vi "PIDPressure2.vi"() -> ()   [LabVIEW 2015]
uses:
  <vilib>/DAQmx/write.llb/DAQmx Write (Digital 1D Bool NChan 1Samp 1Line).vi
  <vilib>/DAQmx/write.llb/DAQmx Write (Digital Bool 1Line 1Point).vi
  <vilib>/DAQmx/read.llb/DAQmx Read (Analog DBL 1Chan 1Samp).vi
  <vilib>/DAQmx/write.llb/DAQmx Write (Analog DBL 1Chan 1Samp).vi
  <vilib>/Analysis/baseanly.llb/Mean (DBL).vi
  <vilib>/DAQmx/read.llb/DAQmx Read (Analog 1D Wfm NChan NSamp).vi
  <vilib>/DAQmx/miscellaneous.llb/DAQmx Fill In Error Info.vi
  <vilib>/addons/control/pid/NI_PID_autopid.lvlib
  <vilib>/Analysis/NI_AALBase.lvlib
panel:
  in  "Manual Control 2":bool
  in  "Heater On/Off":bool
  out "Voltage Reading(Temp)":dbl format="%#_13g"
  out "Temperature (Celcius)":dbl format="%#.1g"
  out "Temp(C)":dbl(slide) scale=-10.0..100.0
  out "Temp Chart":dbl(graph)
  out "Temp Chart 2":dbl(graph)
  out "Temp":dbl
  in  "stop 2":bool
  in  "autotuning parameters 2":T1={"controller type"=1, "relay cycles"=3, "relay amplitude"=1.0, "control specification"=2, "PV noise level"=0.1} {"PV noise level" format="%.2f"; "control specification" items=["normal", "fast", "slow"]; "relay amplitude" format="%.2f"; "controller type" items=["PID", "PI", "P"]}
  in  "PID gains 2":T2={"proportional gain (Kc)"=1.0, "integral time (Ti, min)"=0.01, "derivative time (Td, min)"=0.0} {"derivative time (Td, min)" format="%.3f"; "integral time (Ti, min)" format="%.3f"; "proportional gain (Kc)" format="%.3f"}
  out "PID gains out 2":T2={"proportional gain (Kc)"=1.0, "integral time (Ti, min)"=0.01, "derivative time (Td, min)"=0.0} {"derivative time (Td, min)" format="%.3f"; "integral time (Ti, min)" format="%.3f"; "proportional gain (Kc)" format="%.3f"}
  in  "autotune? (F) 2":bool
  in  "reinitialize? (F) 2":bool
  in  "setpoint in C":dbl format="%.2f"
  out "Control Value Temp":dbl
  out "ms to wait":dbl
  out "Loop 1":i32
  out "Loop 2":i32
  in  "Voltage setting":dbl format="%#_13g"
  in  "Manual Control":bool
  out "Control Value":dbl
  in  "setpoint in Bar":dbl format="%#.5f"
  in  "reinitialize? (F)":bool
  in  "autotune? (F)":bool
  out "PID gains out":T2={"proportional gain (Kc)"=1.0, "integral time (Ti, min)"=0.01, "derivative time (Td, min)"=0.0} {"derivative time (Td, min)" format="%.3f"; "integral time (Ti, min)" format="%.3f"; "proportional gain (Kc)" format="%.3f"}
  in  "PID gains":T2={"proportional gain (Kc)"=1.0, "integral time (Ti, min)"=0.01, "derivative time (Td, min)"=0.0} {"derivative time (Td, min)" format="%.3f"; "integral time (Ti, min)" format="%.3f"; "proportional gain (Kc)" format="%.3f"}
  in  "autotuning parameters":T1={"controller type"=1, "relay cycles"=3, "relay amplitude"=1.0, "control specification"=2, "PV noise level"=0.1} {"PV noise level" format="%.2f"; "control specification" items=["normal", "fast", "slow"]; "relay amplitude" format="%.2f"; "controller type" items=["PID", "PI", "P"]}
  in  "stop":bool
  out "Pressure Chart 2":dbl(graph)
  out "Voltage":dbl(graph)
  out "Pressure":dbl format="%#.3g"
  out "Voltage Reading(pressure)":dbl format="%#_13g"
  # "Readings"
  # "Controls"
  # "PID Settings"
  # "51.12139\n\n0.044676"
  # "Readings"
  # "Controls"
  # "PID Settings"
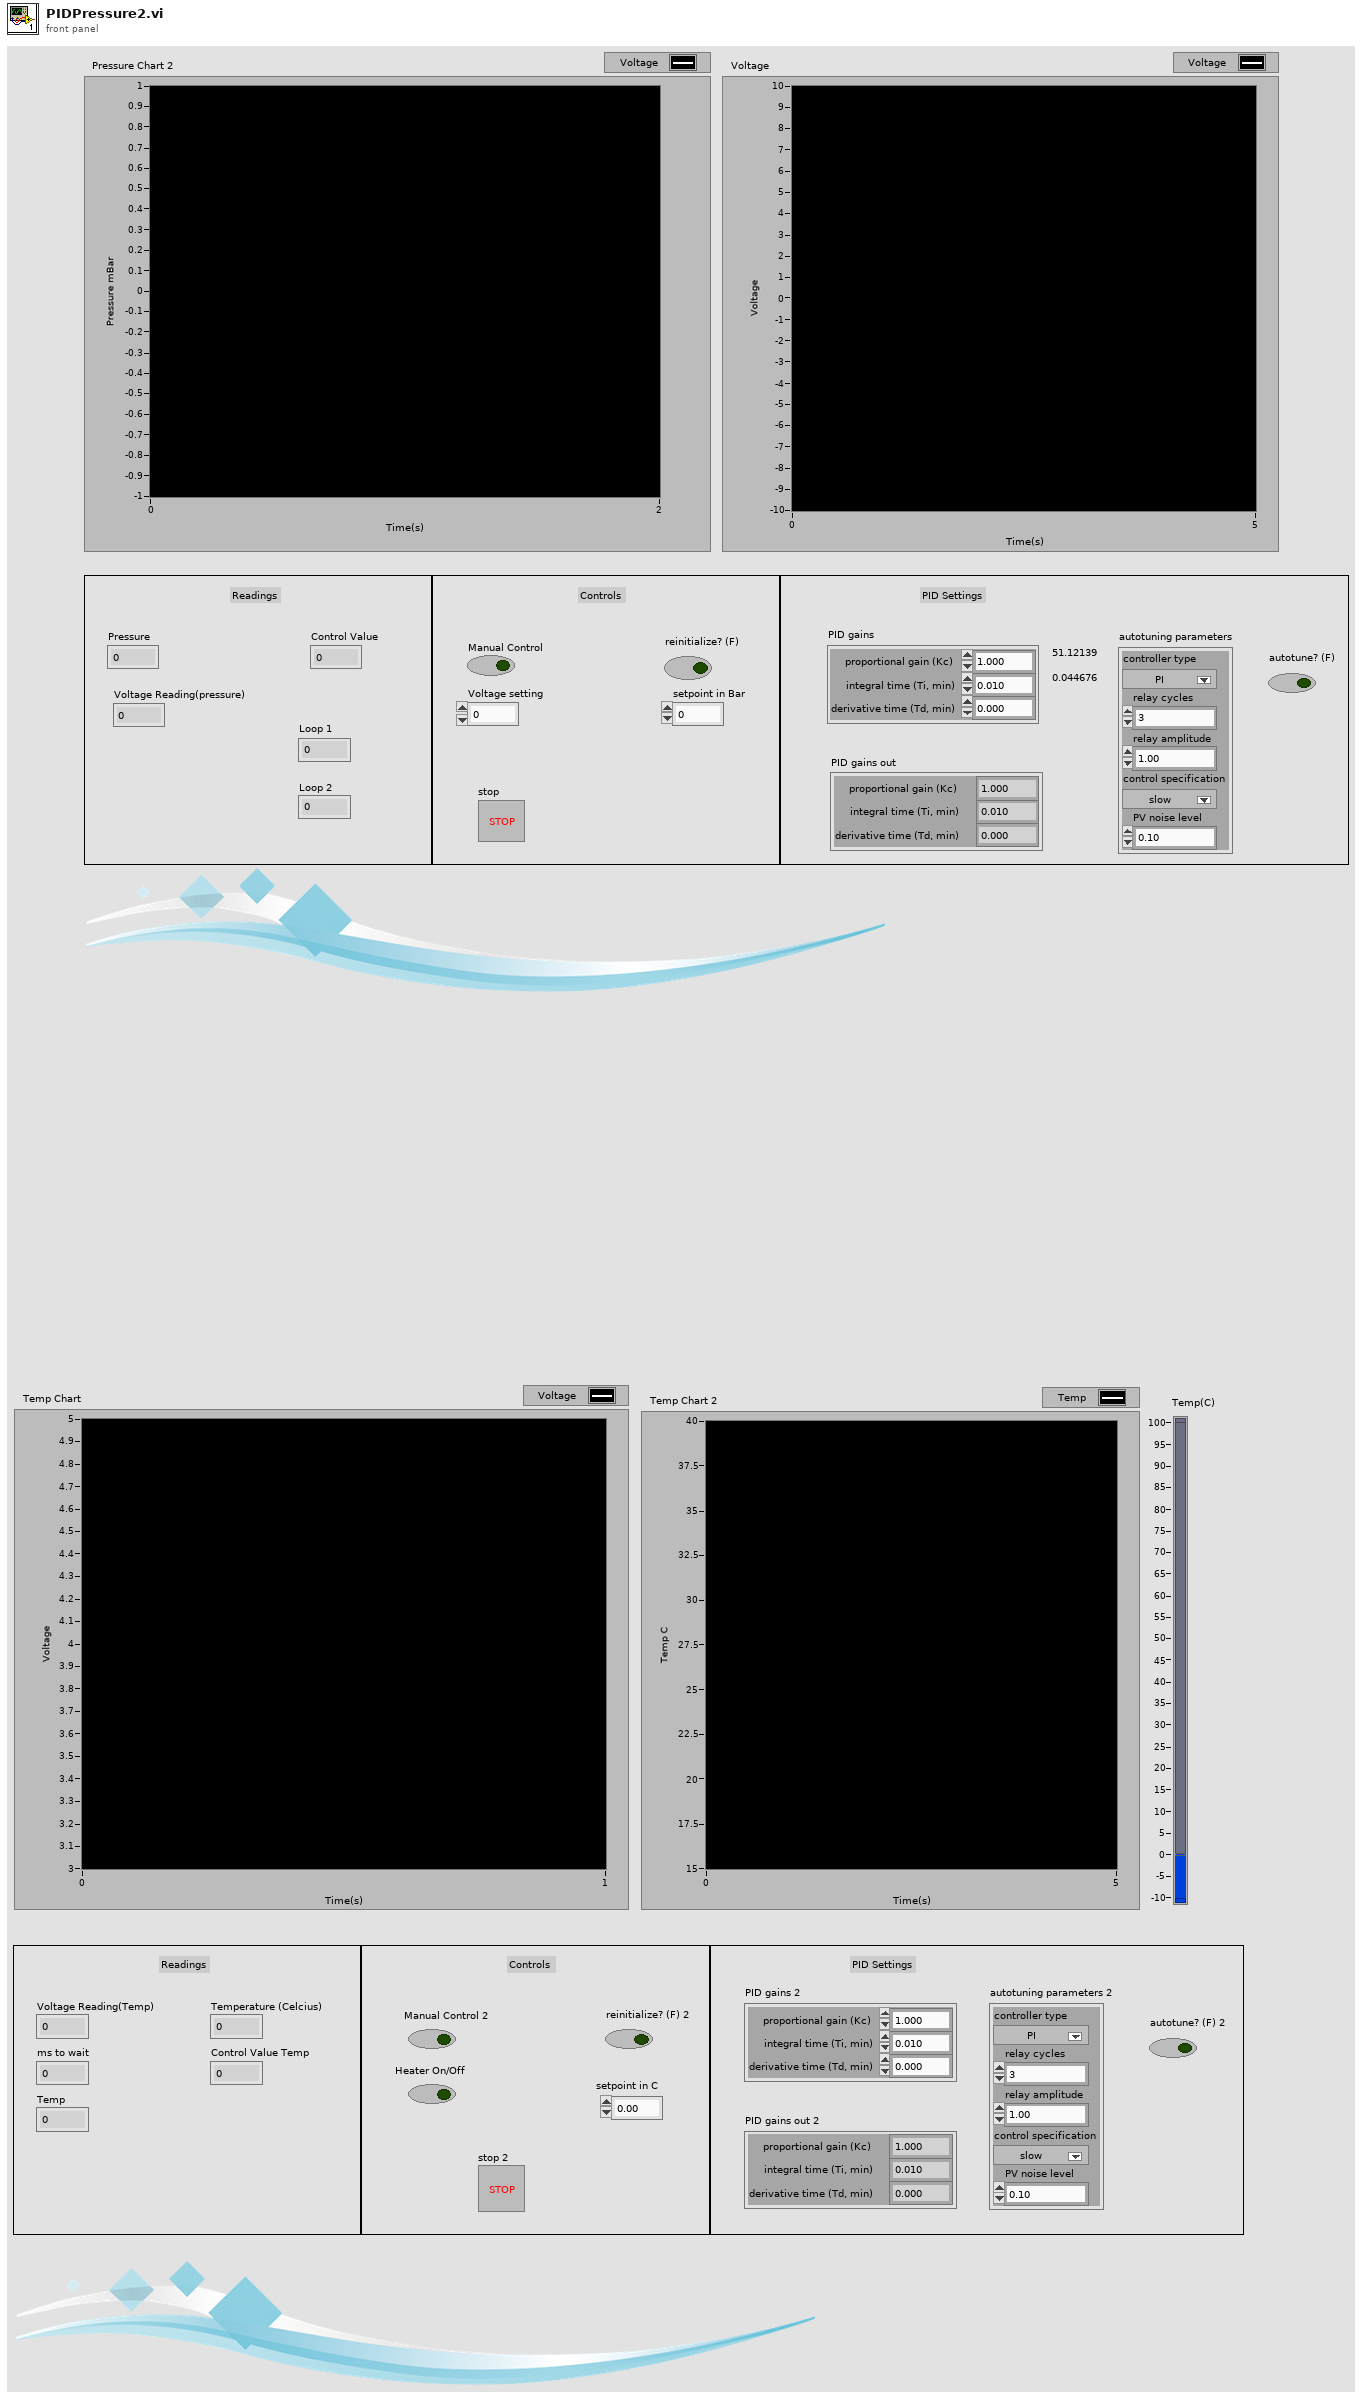
[diagram p1: front panel]
types:
  T1 = cluster{"controller type":u16, "relay cycles":i32, "relay amplitude":dbl, "control specification":u16, "PV noise level":dbl}
  T2 = cluster{"proportional gain (Kc)":dbl, "integral time (Ti, min)":dbl, "derivative time (Td, min)":dbl}
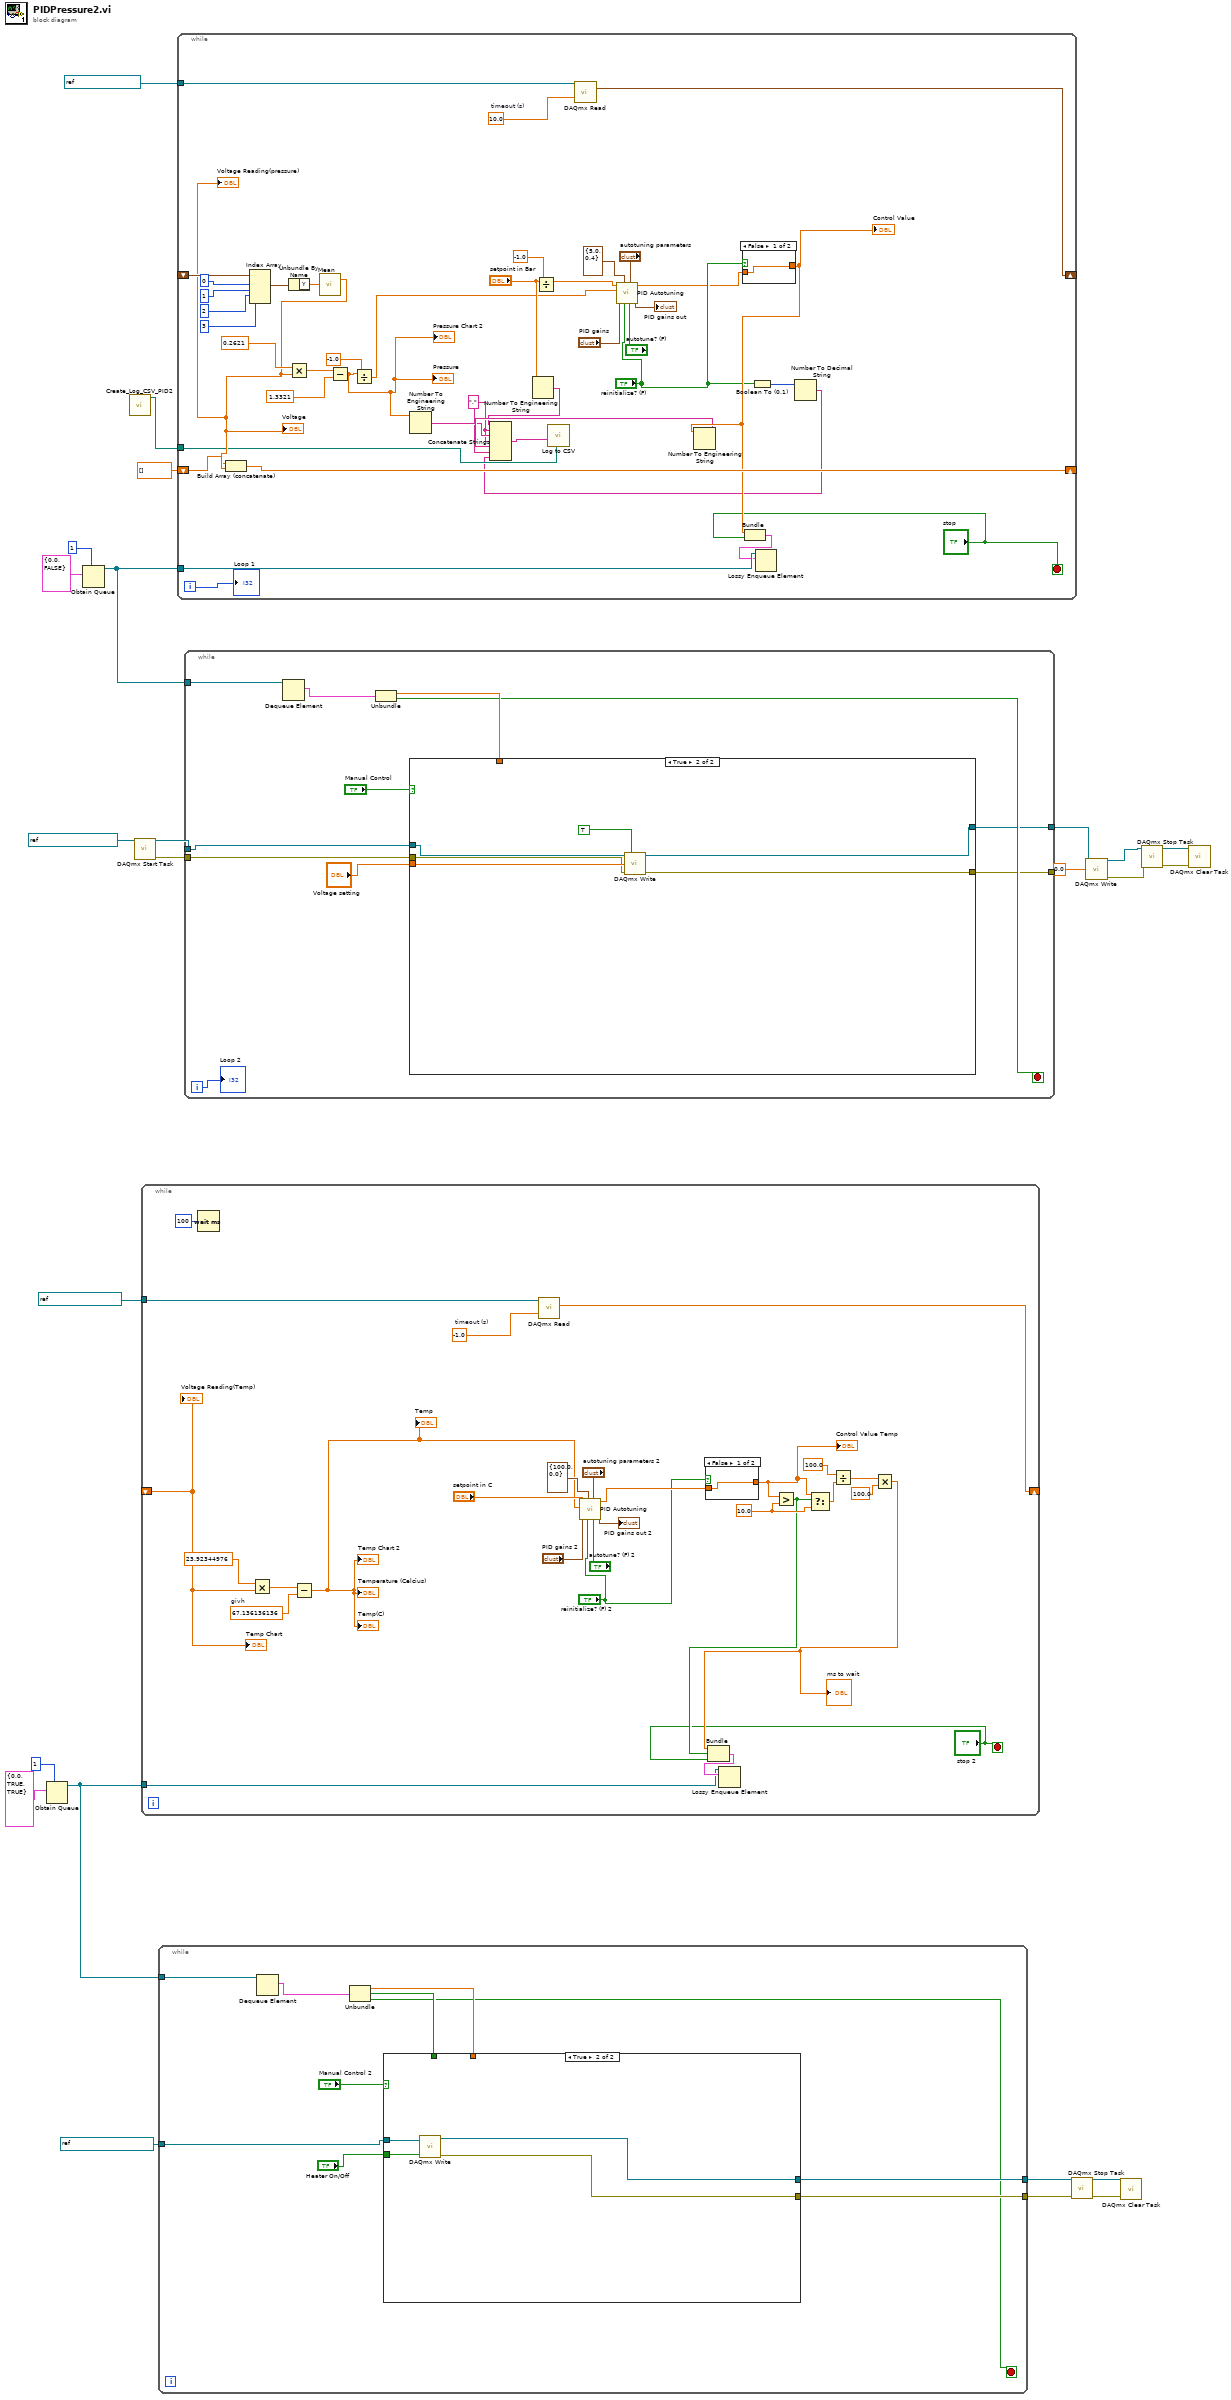
[diagram p0: block diagram]
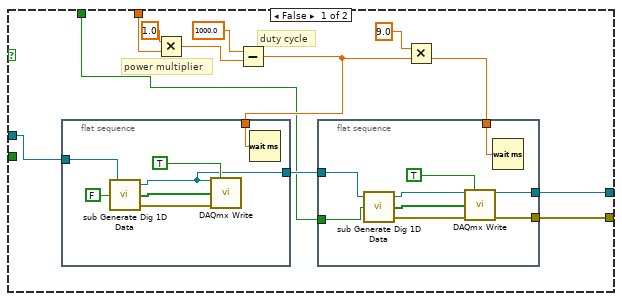
[diagram p2: hidden frame]
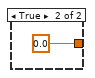
[diagram p3: hidden frame]
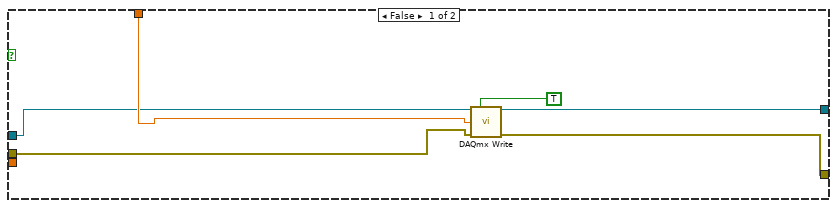
[diagram p4: hidden frame]
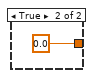
[diagram p5: hidden frame]
diagram:
  n1 = Obtain Queue(max queue size (-1, unlimited)=1, element data type=cluster{dbl, bool, bool} {0.0, TRUE, TRUE}) -> (queue out=w1:refnum<queue>)  [unwired: 3 in, 2 out]
  n2 = Obtain Queue(max queue size (-1, unlimited)=1, element data type=cluster{dbl, bool} {0.0, FALSE}) -> (queue out=w22:refnum<queue>)  [unwired: 3 in, 2 out]
  n3 = call "Create_Log_CSV_PID2.vi"() -> ("path"=w18:path)  [unwired: 11 in]
  n4 = call <vilib>:"DAQmx Start Task.vi"("task/channels in"=refnum<k21> "MyVoltageOutTask") -> ("task out"=w17:refnum<k21>, "error out"=w16:errorcluster)  [unwired: 13 in]
  n5 = while {
    tunnel: refnum<k21> "MyVoltageTask_0" -> [w48]
    shift-right: [w31] -> _
    shift-left: _ -> [w32]
    tunnel: w1 -> [w26]
    stop <- "stop 2" stop-if-true
    w34 = 10.0 ("f")
    w49 = 67.136136136  # givh
    w52 = -1.0  # timeout (s)
    n6 = Wait (ms)(milliseconds to wait=u32 100) -> ()  [unwired: 1 out]
    n7 = Multiply(x=23.92344976, y=w32) -> (x*y=w50:dbl)
    n8 = Subtract(x=w50, y=w49) -> (x-y=w30:dbl)
    "Temperature (Celcius)" <- w30
    "Temp(C)" <- w30
    "Temp Chart 2" <- w30
    "Temp" <- w30
    n9 = call-poly <vilib>:"DAQmx Read.vi"("task/channels in"=w48, "timeout"=w52) -> ("data"=w31:dbl)  [unwired: 11 in, 2 out]
    n10 = call <vilib>:"PID Autotuning.vi"("autotune? (F)"="autotune? (F) 2", "autotuning parameters"="autotuning parameters 2", "reinitialize? (F)"="reinitialize? (F) 2", "output range"=cluster{"output high":dbl, "output low":dbl} {"output high"=100.0, "output low"=0.0}, "PID gains"="PID gains 2", "process variable"=w30, "setpoint"="setpoint in C") -> ("PID gains out"=→"PID gains out 2":T2, "output"=w42:dbl)  [unwired: 1 in, 2 out]
    n11 = case shown="False" "reinitialize? (F) 2" {
      tunnel: [w53 0.0] -> w35
      tunnel: w42 -> [w53 _]
      frame False {
      }
      frame True {
      }
    }
    "Control Value Temp" <- w35
    n12 = Greater?(x=w35, y=w34) -> (0:w28:bool)
    n13 = Select(t=w35, s=w28, f=w34) -> (s? t:f=w36:dbl)
    n14 = Divide(x=100.0, y=w36) -> (x/y=w38:dbl)
    n15 = Multiply(x=w38, y=100.0) -> (x*y=w29:dbl)
    "ms to wait" <- w29
    n16 = Bundle(w29, w28, "stop 2"="stop 2") -> (w27:cluster{dbl, bool, "stop 2":bool})  [unwired: 1 in]
    n17 = Lossy Enqueue Element(queue=w26, element=w27) -> ()  [unwired: 1 in, 4 out]
    "Voltage Reading(Temp)" <- w32
    "Temp Chart" <- w32
  }
  n18 = while {
    tunnel: w1 -> [w64]
    tunnel: refnum<k21> "MyDigitalOutTask_2" -> [w61]
    tunnel: [w57] -> w3
    tunnel: [w56] -> w4
    stop <- w55 stop-if-true
    n19 = Dequeue Element(queue=w64) -> (element=w60:cluster{dbl, bool, bool})  [unwired: 2 in, 3 out]
    n20 = Unbundle(w60) -> (w59:dbl, w58:bool, w55:bool)
    n21 = case shown="True" "Manual Control 2" {
      tunnel: w61 -> [w75 w96]
      tunnel: "Heater On/Off" -> [_ w95]
      tunnel: w59 -> [w74 _]
      tunnel: w58 -> [w69 _]
      tunnel: [w66 w94] -> w57
      tunnel: [w65 w93] -> w56
      frame False {
        # "duty cycle"
        # "power multiplier"
        n22 = flat-sequence {
          tunnel: w75 -> [w89]
          tunnel: [w88] -> w76
          tunnel: w73 -> [w87]
          frame #0 {
            n23 = call <vilib>:"sub Generate Dig 1D Data.vi"("initial value"=FALSE, "task in"=w89) -> ("error out"=w91:errorcluster, "Data"=w92:bool[], "task out"=w88:refnum<k21>)  [unwired: 1 in]
            n24 = call-poly <vilib>:"DAQmx Write.vi"("task/channels in"=w88, "auto start"=TRUE, "data"=w92, "error in"=w91) -> ()  [unwired: 9 in, 3 out]
            n25 = Wait (ms)(milliseconds to wait=w87) -> ()  [unwired: 1 out]
          }
        }
        n26 = Multiply(x=1.0, y=w74) -> (x*y=w68:dbl)
        n27 = Subtract(x=1000.0, y=w68) -> (x-y=w73:dbl)
        n28 = flat-sequence {
          tunnel: w76 -> [w81]
          tunnel: w71 -> [w80]
          tunnel: w69 -> [w79]
          tunnel: [w78] -> w66
          tunnel: [w77] -> w65
          frame #0 {
            n29 = call <vilib>:"sub Generate Dig 1D Data.vi"("initial value"=w79, "task in"=w81) -> ("error out"=w84:errorcluster, "Data"=w82:bool[], "task out"=w83:refnum<k21>)  [unwired: 1 in]
            n30 = call-poly <vilib>:"DAQmx Write.vi"("task/channels in"=w83, "auto start"=TRUE, "data"=w82, "error in"=w84) -> ("task out"=w78:refnum<k21>, "error out"=w77:errorcluster)  [unwired: 9 in, 1 out]
            n31 = Wait (ms)(milliseconds to wait=w80) -> ()  [unwired: 1 out]
          }
        }
        n32 = Multiply(x=9.0, y=w73) -> (x*y=w71:dbl)
      }
      frame True {
        n33 = call-poly <vilib>:"DAQmx Write.vi"("task/channels in"=w96, "data"=w95) -> ("task out"=w94:refnum<k21>, "error out"=w93:errorcluster)  [unwired: 11 in, 1 out]
      }
    }
  }
  n34 = while {
    tunnel: refnum<k21> "MyVoltageTask" -> [w134]
    shift-right: [w128] -> _
    shift-left: _ -> [w121]
    tunnel: w22 -> [w127]
    shift-right: [w116] -> _
    shift-left: dbl[] [] -> [w117]
    tunnel: w18 -> [w110]
    i -> [w102]
    stop <- "stop" stop-if-true
    w105 = ","
    w138 = 10.0  # timeout (s)
    n35 = Index Array(array=w121, index #1=0 ("index"), index #2=1 ("index"), index #3=2 ("index"), index #4=3 ("index")) -> (element #1=w120:waveform(dbl))  [unwired: 3 out]
    n36 = Unbundle By Name(w120) -> ("Y"=w119:dbl[])
    n37 = call-poly <vilib>:"Mean.vi"("X"=w119) -> ("mean"=w118:dbl)  [unwired: 1 out]
    "Voltage Reading(pressure)" <- w118
    "Voltage" <- w118
    n38 = Build Array (concatenate)(w117, w118) -> (w116:dbl[])
    n39 = Multiply(x=0.2621, y=w118) -> (x*y=w136:dbl)
    n40 = Subtract(x=w136, y=1.3321) -> (x-y=w114:dbl)
    "Pressure" <- w114
    "Pressure Chart 2" <- w114
    n41 = Divide(x=w114, y=-1.0) -> (x/y=w100:dbl)
    n42 = Number To Engineering String(4:w114) -> (0:w109:string)  [unwired: 3 in]
    n43 = Number To Engineering String(4:"setpoint in Bar") -> (0:w108:string)  [unwired: 3 in]
    n44 = Divide(x="setpoint in Bar", y=-1.0) -> (x/y=w99:dbl)
    n45 = call-poly <vilib>:"DAQmx Read.vi"("task/channels in"=w134, "timeout"=w138) -> ("data"=w128:waveform(dbl)[])  [unwired: 11 in, 2 out]
    n46 = call <vilib>:"PID Autotuning.vi"("autotune? (F)"="autotune? (F)", "autotuning parameters"="autotuning parameters", "reinitialize? (F)"="reinitialize? (F)", "output range"=cluster{"output high":dbl, "output low":dbl} {"output high"=5.0, "output low"=0.4}, "PID gains"="PID gains", "process variable"=w100, "setpoint"=w99) -> ("PID gains out"=→"PID gains out":T2, "output"=w97:dbl)  [unwired: 1 in, 2 out]
    n47 = case shown="False" "reinitialize? (F)" {
      tunnel: [w139 0.0] -> w113
      tunnel: w97 -> [w139 _]
      frame False {
      }
      frame True {
      }
    }
    "Control Value" <- w113
    n48 = Number To Engineering String(4:w113) -> (0:w112:string)  [unwired: 3 in]
    n49 = Bundle("output"=w113, "stop"="stop") -> (w126:cluster{"output":dbl, "stop":bool})  [unwired: 1 in]
    n50 = Boolean To (0,1)(Boolean="reinitialize? (F)") -> (0, 1=w106:i16)
    n51 = Lossy Enqueue Element(queue=w127, element=w126) -> ()  [unwired: 1 in, 4 out]
    n52 = Number To Decimal String(number=w106) -> (decimal integer string=w104:string)  [unwired: 1 in]
    n53 = Concatenate Strings(w108, w105, w109, w105, w112, w105, w104) -> (w111:string)
    n54 = call "Log to CSV.vi"("Data Str"=w111, "Path"=w110) -> ()  [unwired: 5 in, 1 out]
    "Loop 1" <- w102
  }
  n55 = while {
    tunnel: w22 -> [w151]
    tunnel: w17 -> [w149]
    tunnel: [w143] -> w14
    tunnel: w16 -> [w142]
    tunnel: [w141] -> _
    i -> [w145]
    stop <- w144 stop-if-true
    n56 = Dequeue Element(queue=w151) -> (element=w148:cluster{dbl, bool})  [unwired: 2 in, 3 out]
    n57 = Unbundle(w148) -> (w147:dbl, w144:bool)
    n58 = case shown="True" "Manual Control" {
      tunnel: w149 -> [w155 w162]
      tunnel: w147 -> [w156 _]
      tunnel: "Voltage setting" -> [_ w161]
      tunnel: [w154 w160] -> w143
      tunnel: w142 -> [w153 w159]
      tunnel: [w152 w158] -> w141
      frame False {
        n59 = call-poly <vilib>:"DAQmx Write.vi"("task/channels in"=w155, "auto start"=TRUE, "data"=w156, "error in"=w153) -> ("task out"=w154:refnum<k21>, "error out"=w152:errorcluster)  [unwired: 9 in, 1 out]
      }
      frame True {
        n60 = call-poly <vilib>:"DAQmx Write.vi"("task/channels in"=w162, "auto start"=TRUE, "data"=w161, "error in"=w159) -> ("task out"=w160:refnum<k21>, "error out"=w158:errorcluster)  [unwired: 9 in, 1 out]
      }
    }
    "Loop 2" <- w145
  }
  n61 = call <vilib>:"DAQmx Stop Task.vi"("task/channels in"=w3, "error in"=w4) -> ("task out"=w5:refnum<k21>, "error out"=w6:errorcluster)  [unwired: 12 in]
  n62 = call-poly <vilib>:"DAQmx Write.vi"("task/channels in"=w14, "data"=0.0) -> ("task out"=w13:refnum<k21>, "error out"=w12:errorcluster)  [unwired: 11 in, 1 out]
  n63 = call <vilib>:"DAQmx Clear Task.vi"("task in"=w5, "error in"=w6) -> ()  [unwired: 13 in, 1 out]
  n64 = call <vilib>:"DAQmx Stop Task.vi"("task/channels in"=w13, "error in"=w12) -> ("task out"=w15:refnum<k21>, "error out"=w11:errorcluster)  [unwired: 12 in]
  n65 = call <vilib>:"DAQmx Clear Task.vi"("task in"=w15, "error in"=w11) -> ()  [unwired: 13 in, 1 out]
